vi "updateColumnHeaders.vi"(8 "error in (no error)":errorcluster, 11 "InputDataLogger in":refnum<class "TestDataLog.lvclass">) -> (0 "error out":errorcluster, 3 "InputDataLogger out":refnum<class "TestDataLog.lvclass">)   [LabVIEW 2015, in "TestDataLog.lvclass"]
uses:
  TestDataLog.lvclass
  <userlib>/Common/Log/Log/Log.lvclass/Log.ctl
  <userlib>/Common/Log/Log/Log.lvclass
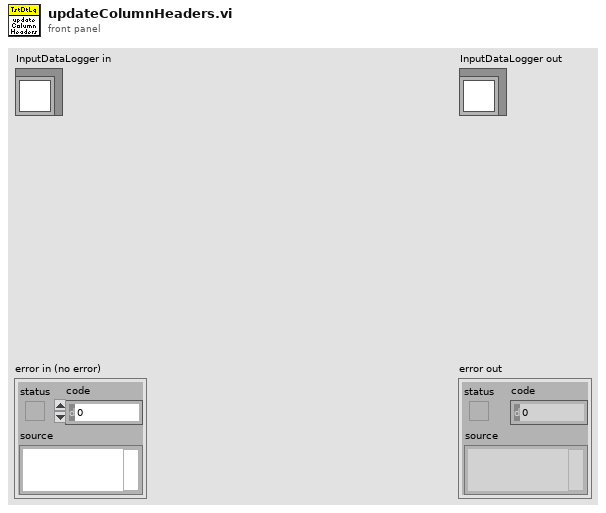
[diagram p1: front panel]
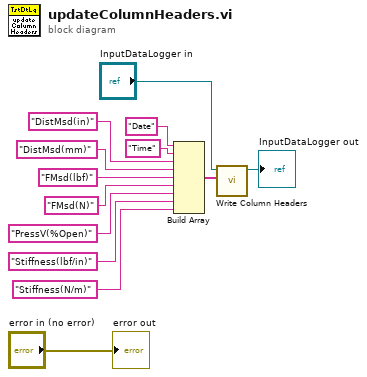
[diagram p0: block diagram]
diagram:
  n1 = Build Array("Date" ("element"), "Time", "DistMsd(in)", "DistMsd(mm)", "FMsd(lbf)", "FMsd(N)", "PressV(%Open)", "Stiffness(lbf/in)", "Stiffness(N/m)") -> (w11:string[])
  n2 = call <userlib>:"Write Column Headers.vi"("Column Headers"=w11, "Logger in"="InputDataLogger in") -> ("Logger out"=→"InputDataLogger out":refnum<class "TestDataLog.lvclass">)  [unwired: 9 in]
  "error out" <- "error in (no error)"
